vi "DataHeader.vi"() -> ()   [LabVIEW 2013]
panel:
  in  "APD/TPos Num":u32
  in  "Save Trap Pos. Data":bool
  in  "Save APD Data\nwith Trap Data":bool
  in  "Start":bool
  in  "BD Frqs":dbl[](array[numeric])
  in  "Data Period (s)":dbl
  in  "Channel Pattern":dbl
  in  "N Channels":dbl
  in  "Data Type":u32
  out "N sets should be saved (MCL)":dbl=160.0 caption="N sets should be saved"
  in  "Fast Scan Dir":bool=TRUE
  in  "Scan Range (V)\n(of steps)":dbl=3.5
  in  "Scan steps (x)":u64=40
  out "Cycles/step (MCL)":u64=2000 caption="Cycles/step" format="%.0p"
  in  "Number of scans (MCL)":u64=1 caption="Scans"
  out "Initial X":dbl=1.6310662274449115
  out "Initial Y":dbl=2.5691326639606933
  in  "2D or 1D Scan":bool=TRUE
  in  "Scan lines (y)":u64=20
  out "N sets should be saved":dbl=133.2
  in  "Scan BD":bool=TRUE
  out "Scan Range (MHz)":dbl=-10.0
  out "Scan steps (AOD)":u64=2000
  out "Cycles/step (AOD)":u64=666 format="%.3p"
  in  "Number of F/B Scans (AOD)":u16=1 min=1
  in  "Save ave N":dbl=500.0 caption="Averaging Factor"
  out "Calibrating Trap...":bool
  in  "Cal sets to save":u32=50 min=1 step=1
  in  "N sets to save":u32=200 caption="N Sets"
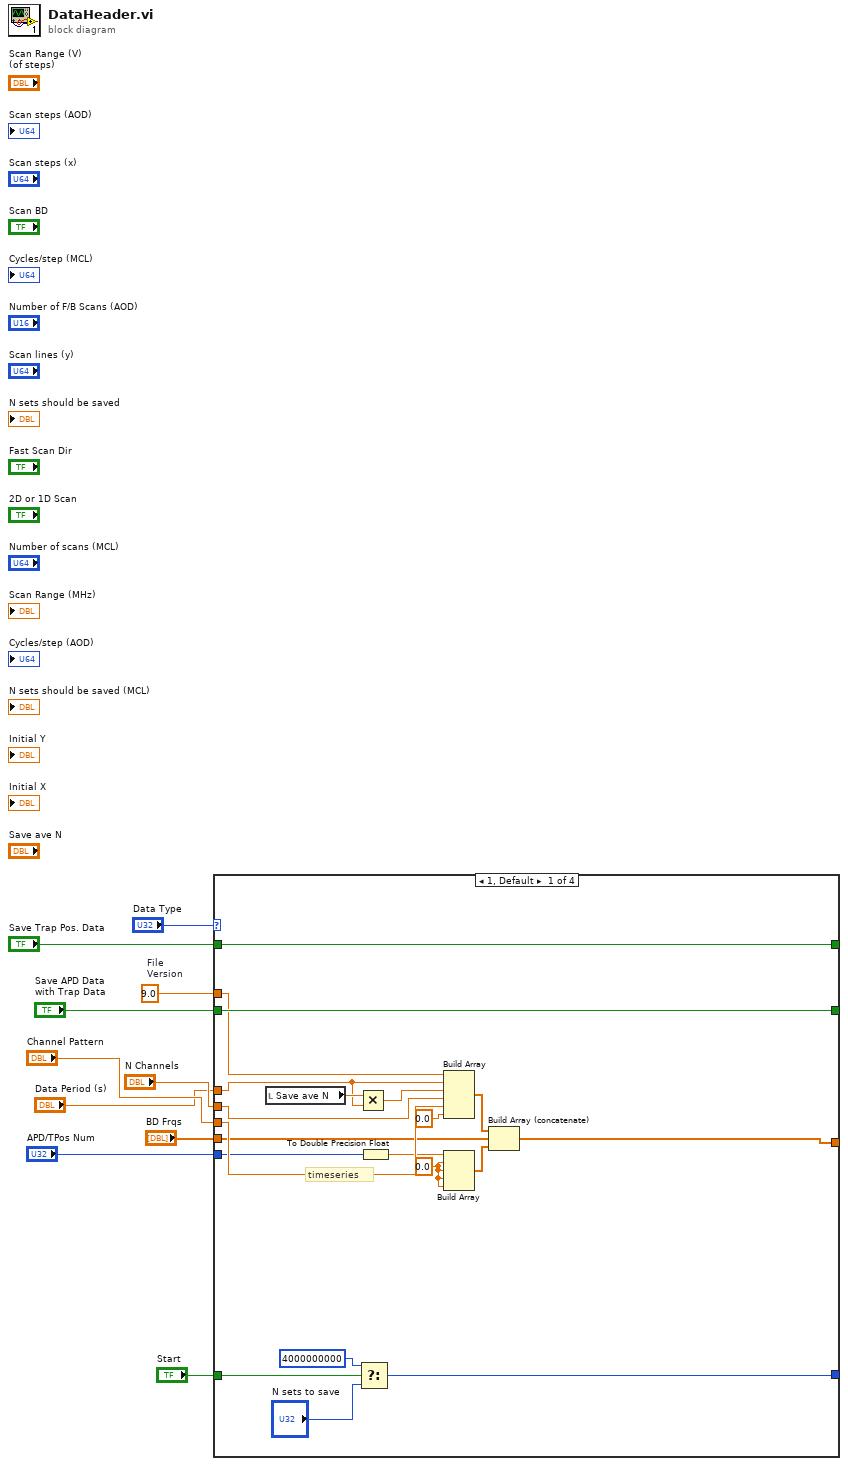
[diagram p0: block diagram]
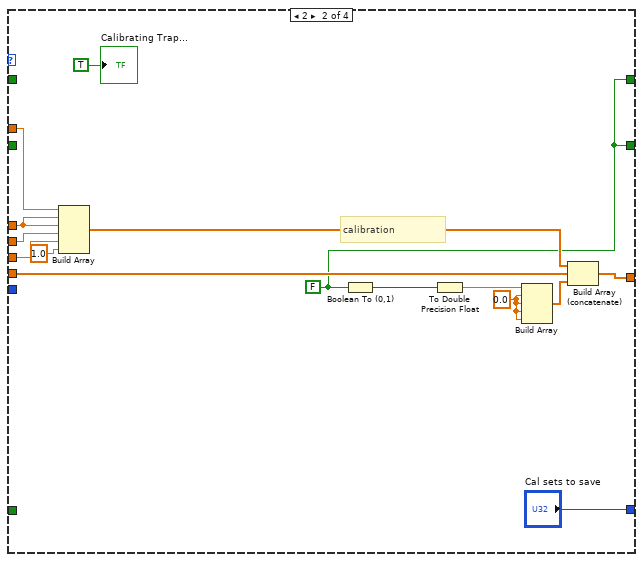
[diagram p2: hidden frame]
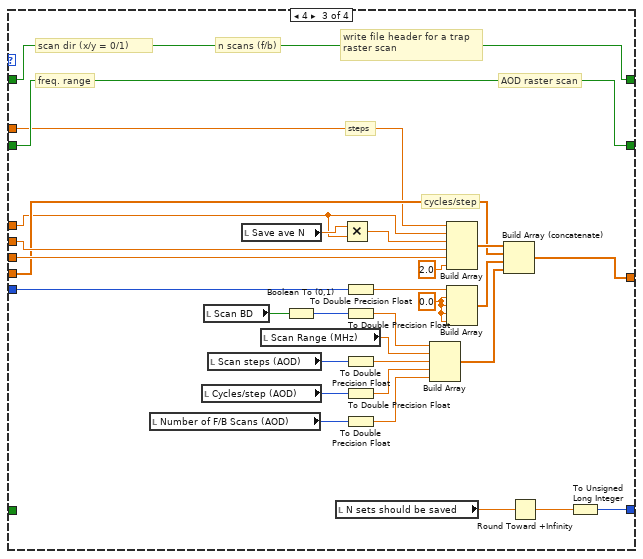
[diagram p3: hidden frame]
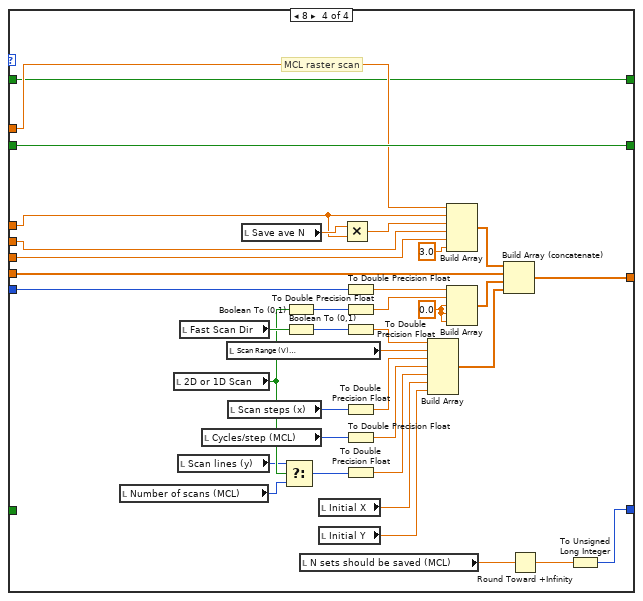
[diagram p4: hidden frame]
diagram:
  w10 = 9.0  # File Version
  n1 = case shown="1, Default" "Data Type" {
    tunnel: "Data Period (s)" -> [w23 w37 w53 w91]
    tunnel: "N Channels" -> [w28 w44 w73 w110]
    tunnel: "Channel Pattern" -> [w27 w43 w72 w109]
    tunnel: [w24 w39 w64 w101] -> _
    tunnel: [w15 "Cal sets to save" w54 w92] -> _
    tunnel: "BD Frqs" -> [w25 w40 w66 w103]
    tunnel: "Save APD Data\nwith Trap Data" -> [w22 _ w50 w89]
    tunnel: [w22 w31 w50 w89] -> _
    tunnel: w10 -> [w18 w32 w48 w87]
    tunnel: "Start" -> [w17 _ _ _]
    tunnel: [w12 w31 w47 w77] -> _
    tunnel: "Save Trap Pos. Data" -> [w12 _ w47 w77]
    tunnel: "APD/TPos Num" -> [w11 _ w46 w76]
    frame 1, Default {
      w13 = 0.0 ("f")
      # "timeseries"
      n2 = local read "Save ave N"() -> (w30:dbl)
      n3 = Multiply(x=w30, y=w23) -> (x*y=w29:dbl)
      n4 = Select(t=u32 4000000000, s=w17, f="N sets to save") -> (s? t:f=w15:u32)
      n5 = To Double Precision Float(number=w11) -> (double precision float=w21:dbl)
      n6 = Build Array(w18, w23, w29, w28, w27, 0.0 ("f")) -> (w26:dbl[])
      n7 = Build Array(w21, w13, w13, w13, w13) -> (w19:dbl[])
      n8 = Build Array (concatenate)(w26, w25, w19) -> (w24:dbl[])
    }
    frame 2 {
      w34 = 0.0 ("f")
      w31 = FALSE ("Save APD Data\nwith Trap Data")
      # "calibration"
      n9 = Build Array(w32, w37, w37, w44, w43, 1.0 ("t")) -> (w41:dbl[])
      n10 = Boolean To (0,1)(Boolean=w31) -> (0, 1=w36:i16)
      n11 = To Double Precision Float(number=w36) -> (double precision float=w35:dbl)
      n12 = Build Array(w35, w34, w34, w34, w34) -> (w33:dbl[])
      n13 = Build Array (concatenate)(w41, w40, w33) -> (w39:dbl[])
      "Calibrating Trap..." <- TRUE ("Calibrating...")
    }
    frame 4 {
      w51 = 0.0 ("f")
      # "write file header for a trap \nraster scan"
      # "scan dir (x/y = 0/1)"
      # "cycles/step"
      # "n scans (f/b)"
      # "steps"
      # "freq. range"
      # "AOD raster scan"
      n14 = local read "Number of F/B Scans (AOD)"() -> (w58:u16)
      n15 = local read "Cycles/step (AOD)"() -> (w60:u64)
      n16 = local read "Scan BD"() -> (w70:bool)
      n17 = local read "Scan steps (AOD)"() -> (w62:u64)
      n18 = local read "Save ave N"() -> (w75:dbl)
      n19 = local read "Scan Range (MHz)"() -> (w63:dbl)
      n20 = Boolean To (0,1)(Boolean=w70) -> (0, 1=w69:i16)
      n21 = local read "N sets should be saved"() -> (w55:dbl)
      n22 = Multiply(x=w75, y=w53) -> (x*y=w74:dbl)
      n23 = To Double Precision Float(number=w46) -> (double precision float=w52:dbl)
      n24 = To Double Precision Float(number=w69) -> (double precision float=w68:dbl)
      n25 = To Double Precision Float(number=w62) -> (double precision float=w61:dbl)
      n26 = To Double Precision Float(number=w60) -> (double precision float=w59:dbl)
      n27 = To Double Precision Float(number=w58) -> (double precision float=w57:dbl)
      n28 = Build Array(w68, w63, w61, w59, w57) -> (w65:dbl[])
      n29 = Build Array(w48, w53, w74, w73, w72, 2.0 ("t")) -> (w67:dbl[])
      n30 = Build Array(w52, w51, w51, w51, w51) -> (w49:dbl[])
      n31 = Build Array (concatenate)(w67, w66, w49, w65) -> (w64:dbl[])
      n32 = Round Toward +Infinity(x=w55) -> (ceil(x): smallest int >= x=w56:dbl)
      n33 = To Unsigned Long Integer(number=w56) -> (unsigned 32bit integer=w54:u32)
    }
    frame 8 {
      w84 = 0.0 ("f")
      # "MCL raster scan"
      n34 = local read "Number of scans (MCL)"() -> (w79:u64)
      n35 = local read "2D or 1D Scan"() -> (w81:bool)
      n36 = local read "Scan lines (y)"() -> (w78:u64)
      n37 = local read "Fast Scan Dir"() -> (w107:bool)
      n38 = local read "Cycles/step (MCL)"() -> (w97:u64)
      n39 = local read "Scan Range (V)\n(of steps)"() -> (w100:dbl)
      n40 = local read "Scan steps (x)"() -> (w99:u64)
      n41 = local read "Save ave N"() -> (w112:dbl)
      n42 = Select(t=w78, s=w81, f=w79) -> (s? t:f=w80:u64)
      n43 = Boolean To (0,1)(Boolean=w81) -> (0, 1=w83:i16)
      n44 = Boolean To (0,1)(Boolean=w107) -> (0, 1=w106:i16)
      n45 = local read "N sets should be saved (MCL)"() -> (w93:dbl)
      n46 = local read "Initial X"() -> (w86:dbl)
      n47 = local read "Initial Y"() -> (w85:dbl)
      n48 = Multiply(x=w112, y=w91) -> (x*y=w111:dbl)
      n49 = To Double Precision Float(number=w76) -> (double precision float=w90:dbl)
      n50 = To Double Precision Float(number=w83) -> (double precision float=w82:dbl)
      n51 = To Double Precision Float(number=w106) -> (double precision float=w105:dbl)
      n52 = To Double Precision Float(number=w99) -> (double precision float=w98:dbl)
      n53 = To Double Precision Float(number=w97) -> (double precision float=w96:dbl)
      n54 = To Double Precision Float(number=w80) -> (double precision float=w95:dbl)
      n55 = Build Array(w105, w100, w98, w96, w95, w86, w85) -> (w102:dbl[])
      n56 = Build Array(w87, w91, w111, w110, w109, 3.0 ("t")) -> (w104:dbl[])
      n57 = Build Array(w90, w82, w84, w84, w84) -> (w88:dbl[])
      n58 = Build Array (concatenate)(w104, w103, w88, w102) -> (w101:dbl[])
      n59 = Round Toward +Infinity(x=w93) -> (ceil(x): smallest int >= x=w94:dbl)
      n60 = To Unsigned Long Integer(number=w94) -> (unsigned 32bit integer=w92:u32)
    }
  }
